vi "Decode.vi"(8 "error in (no error)":errorcluster, 10 "Binary string in":string, 11 "obj in":refnum<class "Gaze.lvclass">) -> (0 "error out":errorcluster, 1 "Data out":refnum<class "Data.lvclass">, 2 "Rest of binary string":string, 3 "obj out":refnum<class "Gaze.lvclass">)   [LabVIEW 2020, in "Gaze.lvclass"]
uses:
  Gaze.lvclass
  Data Class/Data.lvclass
  Data Class/Datatypes/Data_Gaze_class/Attribute.vi
  Gaze.lvclass/Gaze.ctl
  Data Class/Datatypes/Data_Gaze_class/Data_Gaze.lvclass
  C:/Users/theod/Desktop/API - EyeT data streaming to IC/Smart Eye API/Source/Classes/Smart Eye Pro Drivers/Data Class/Data.lvclass
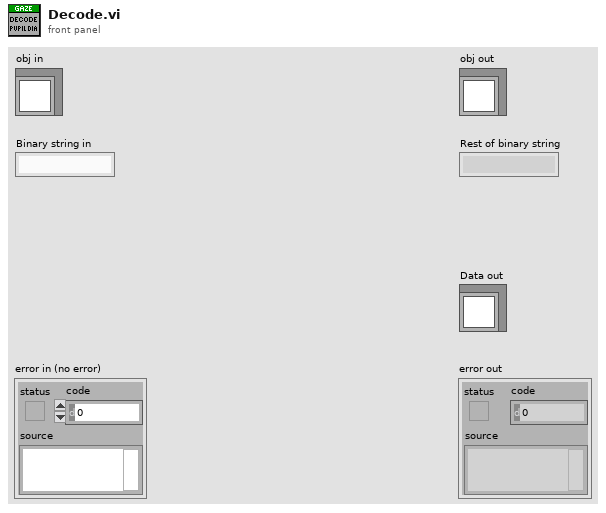
[diagram p1: front panel]
types:
  T1 = typedef "Data_Gaze.lvclass/Attribute.vi" = cluster{"EyePosition":dbl[], "GazeDirection":dbl[], "LeftGazeDirectionQ":dbl, "RightGazeDirectionQ":dbl, "GazeHeading":dbl, "GazePitch":dbl, "LeftGazeHeading":dbl, "LeftGazePitch":dbl, "RightGazeHeading":dbl, "RightGazePitch":dbl}
  T2 = enum16{"big-endian, network order", "native, host order", "little-endian"}
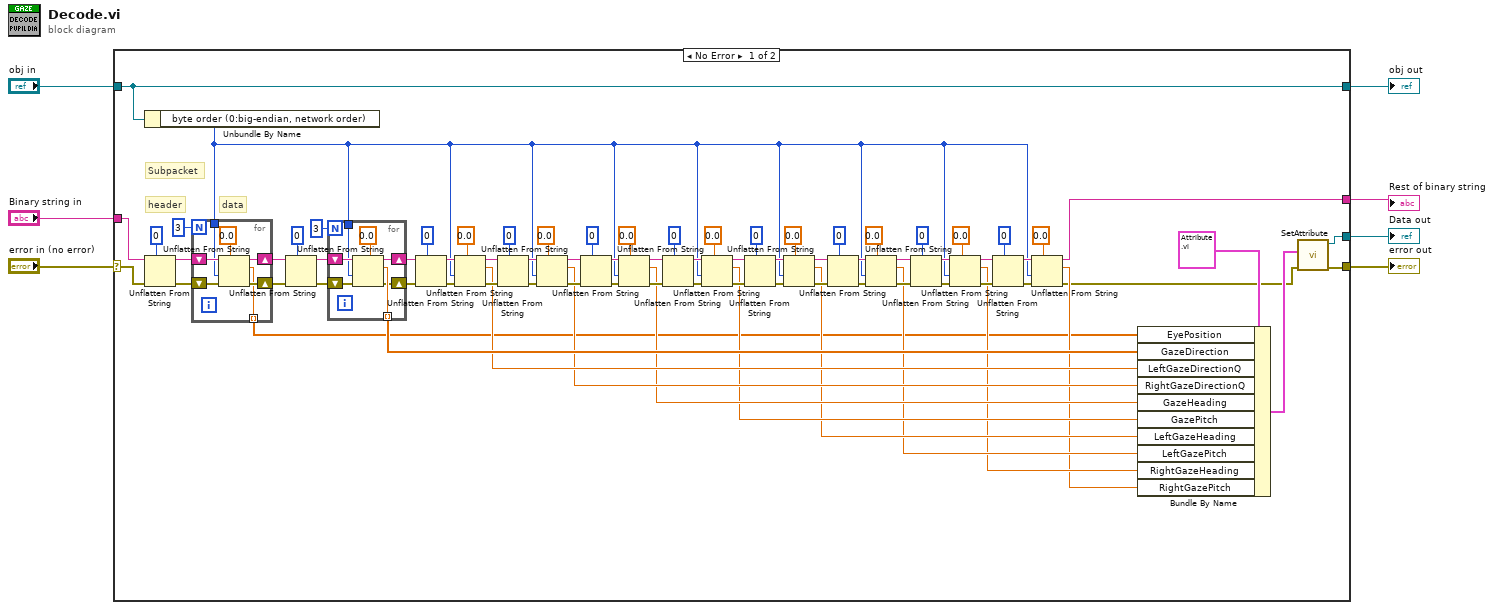
[diagram p0: block diagram]
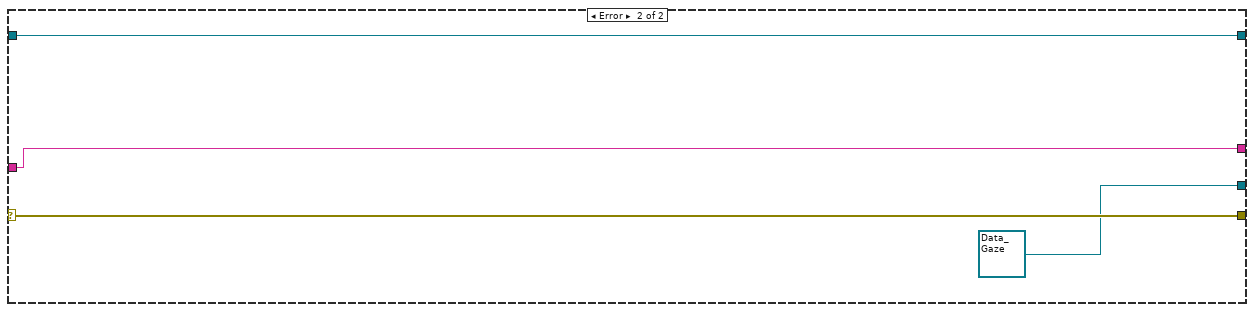
[diagram p2: hidden frame]
diagram:
  n1 = case shown="No Error" "error in (no error)" {
    selector: "error in (no error)" -> [w21 w103]
    tunnel: [w83 w103] -> w6
    tunnel: "obj in" -> [w9 w102]
    tunnel: [w9 w102] -> w4
    tunnel: "Binary string in" -> [w20 w100]
    tunnel: [w82 refnum<class "Data_Gaze.lvclass"> refnum ("Data_Pupil_Diameter")] -> w2
    tunnel: [w19 w100] -> w1
    frame No Error {
      # "header"
      # "data"
      # "Subpacket"
      n2 = Unbundle By Name(w9) -> ("byte order (0:big-endian, network order)"=w8:T2)
      n3 = Unflatten From String(type=u32 0, binary string=w20, error in (no error)=w21) -> (rest of the binary string=w13:string, error out=w11:errorcluster)  [unwired: 2 in, 1 out]
      n4 = for {
        N: 3 -> [_]
        tunnel: [w90] -> w18 mode=indexing
        shift-right: [w92] -> w81
        shift-left: w13 -> [w89]
        shift-right: [w91] -> w77
        shift-left: w11 -> [w88]
        tunnel: w8 -> [w86]
        n5 = Unflatten From String(type=0.0, binary string=w89, byte order (0:big-endian, network order)=w86, error in (no error)=w88) -> (rest of the binary string=w92:string, value=w90:dbl, error out=w91:errorcluster)  [unwired: 1 in]
      }
      n6 = Unflatten From String(type=u32 0, binary string=w81, error in (no error)=w77) -> (rest of the binary string=w17:string, error out=w15:errorcluster)  [unwired: 2 in, 1 out]
      n7 = for {
        N: 3 -> [_]
        tunnel: [w98] -> w32 mode=indexing
        shift-right: [w99] -> w35
        shift-left: w17 -> [w96]
        shift-right: [w97] -> w23
        shift-left: w15 -> [w95]
        tunnel: w8 -> [w93]
        n8 = Unflatten From String(type=0.0, binary string=w96, byte order (0:big-endian, network order)=w93, error in (no error)=w95) -> (rest of the binary string=w99:string, value=w98:dbl, error out=w97:errorcluster)  [unwired: 1 in]
      }
      n9 = Unflatten From String(type=0, binary string=w35, error in (no error)=w23) -> (rest of the binary string=w75:string, error out=w34:errorcluster)  [unwired: 2 in, 1 out]
      n10 = Unflatten From String(type=0.0, binary string=w75, byte order (0:big-endian, network order)=w8, error in (no error)=w34) -> (rest of the binary string=w73:string, value=w31:dbl, error out=w33:errorcluster)  [unwired: 1 in]
      n11 = Unflatten From String(type=u32 0, binary string=w73, error in (no error)=w33) -> (rest of the binary string=w80:string, error out=w76:errorcluster)  [unwired: 2 in, 1 out]
      n12 = Unflatten From String(type=0.0, binary string=w80, byte order (0:big-endian, network order)=w8, error in (no error)=w76) -> (rest of the binary string=w68:string, value=w30:dbl, error out=w66:errorcluster)  [unwired: 1 in]
      n13 = Unflatten From String(type=u32 0, binary string=w68, error in (no error)=w66) -> (rest of the binary string=w72:string, error out=w69:errorcluster)  [unwired: 2 in, 1 out]
      n14 = Unflatten From String(type=0.0, binary string=w72, byte order (0:big-endian, network order)=w8, error in (no error)=w69) -> (rest of the binary string=w47:string, value=w29:dbl, error out=w45:errorcluster)  [unwired: 1 in]
      n15 = Unflatten From String(type=0, binary string=w47, error in (no error)=w45) -> (rest of the binary string=w62:string, error out=w44:errorcluster)  [unwired: 2 in, 1 out]
      n16 = Unflatten From String(type=0.0, binary string=w62, byte order (0:big-endian, network order)=w8, error in (no error)=w44) -> (rest of the binary string=w60:string, value=w28:dbl, error out=w43:errorcluster)  [unwired: 1 in]
      n17 = Unflatten From String(type=u32 0, binary string=w60, error in (no error)=w43) -> (rest of the binary string=w65:string, error out=w42:errorcluster)  [unwired: 2 in, 1 out]
      n18 = Unflatten From String(type=0.0, binary string=w65, byte order (0:big-endian, network order)=w8, error in (no error)=w42) -> (rest of the binary string=w56:string, value=w27:dbl, error out=w41:errorcluster)  [unwired: 1 in]
      n19 = Unflatten From String(type=u32 0, binary string=w56, error in (no error)=w41) -> (rest of the binary string=w59:string, error out=w40:errorcluster)  [unwired: 2 in, 1 out]
      n20 = Unflatten From String(type=0.0, binary string=w59, byte order (0:big-endian, network order)=w8, error in (no error)=w40) -> (rest of the binary string=w46:string, value=w26:dbl, error out=w39:errorcluster)  [unwired: 1 in]
      n21 = Unflatten From String(type=0, binary string=w46, error in (no error)=w39) -> (rest of the binary string=w51:string, error out=w38:errorcluster)  [unwired: 2 in, 1 out]
      n22 = Unflatten From String(type=0.0, binary string=w51, byte order (0:big-endian, network order)=w8, error in (no error)=w38) -> (rest of the binary string=w53:string, value=w25:dbl, error out=w37:errorcluster)  [unwired: 1 in]
      n23 = Unflatten From String(type=u32 0, binary string=w53, error in (no error)=w37) -> (rest of the binary string=w48:string, error out=w36:errorcluster)  [unwired: 2 in, 1 out]
      n24 = Unflatten From String(type=0.0, binary string=w48, byte order (0:big-endian, network order)=w8, error in (no error)=w36) -> (rest of the binary string=w19:string, value=w24:dbl, error out=w22:errorcluster)  [unwired: 1 in]
      n25 = Bundle By Name(cluster=T1 {"EyePosition"=[], "GazeDirection"=[], "LeftGazeDirectionQ"=0.0, "RightGazeDirectionQ"=0.0, "GazeHeading"=0.0, "GazePitch"=0.0, "LeftGazeHeading"=0.0, "LeftGazePitch"=0.0, "RightGazeHeading"=0.0, "RightGazePitch"=0.0} ("Attribute"), "EyePosition"=w18, "GazeDirection"=w32, "LeftGazeDirectionQ"=w31, "RightGazeDirectionQ"=w30, "GazeHeading"=w29, "GazePitch"=w28, "LeftGazeHeading"=w27, "LeftGazePitch"=w26, "RightGazeHeading"=w25, "RightGazePitch"=w24) -> (w84:T1)
      n26 = call "SetAttribute.vi"("error in (no error)"=w22, "Set Attribute"=w84) -> ("error out"=w83:errorcluster, "Data_Gaze out"=w82:refnum<class "Data_Gaze.lvclass">)  [unwired: 8 in]
    }
    frame Error {
    }
  }
  "error out" <- w6
  "obj out" <- w4
  "Data out" <- w2
  "Rest of binary string" <- w1
